vi "create_channels_DI.vi"(0 "task in":refnum<k21>, 11 "error in":errorcluster) -> (4 "task out":refnum<k21>, 15 "error out":errorcluster)   [LabVIEW 2016]
uses:
  <vilib>/DAQmx/create/channels.llb/DAQmx Create Channel (DO-Digital Output).vi
panel:
  in  "labels":string[](array[string])=["DI Lick"] caption="Labels"
  in  "ports":tag[][](array[tag])=[["Dev1/port1/line1", "Dev1/port2/line5", "Dev1/port0/line17", "Dev1/port0/line29"]]
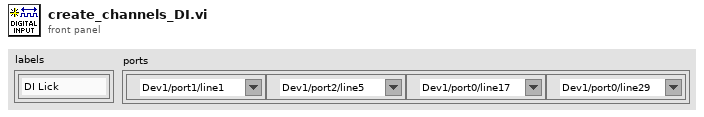
[diagram p1: front panel]
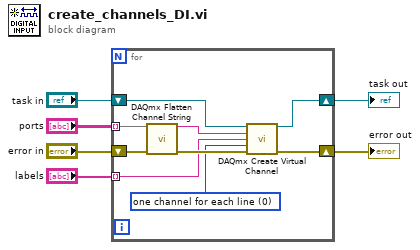
[diagram p0: block diagram]
diagram:
  n1 = for {
    shift-right: [w11] -> w1
    shift-left: "task in" -> [w15]
    shift-right: [w10] -> w4
    shift-left: "error in" -> [w13]
    tunnel: "ports" -> [w8] mode=indexing
    tunnel: "labels" -> [w7] mode=indexing
    w9 = 0 items=["one channel for each line", "one channel for all lines"] ("line grouping")
    n2 = call <vilib>:"DAQmx Flatten Channel String.vi"("names in"=w8, "error in"=w13) -> ("names out"=w14:string, "error out"=w12:errorcluster)  [unwired: 12 in]
    n3 = call-poly <vilib>:"DAQmx Create Virtual Channel.vi"("task in"=w15, "lines"=w14, "name to assign"=w7, "line grouping"=w9, "error in"=w12) -> ("task out"=w11:refnum<k21>, "error out"=w10:errorcluster)  [unwired: 9 in]
  }
  "task out" <- w1
  "error out" <- w4
